vi "Get Name.vi"(8 "error in (no error)":errorcluster, 11 "Release in":refnum<class "Release.lvclass">) -> (0 "error out":errorcluster, 2 "Command Name":string, 3 "Release out":refnum<class "Release.lvclass">)   [LabVIEW 2014, in "Grabber.lvlib" / "Release.lvlib" / "Release.lvclass"]
uses:
  Release.lvclass
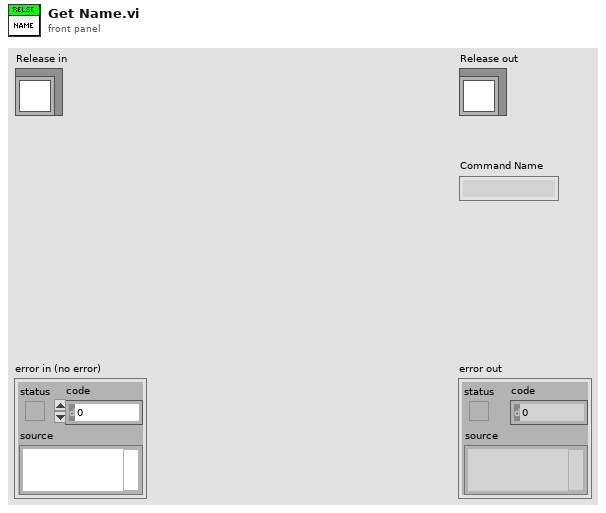
[diagram p1: front panel]
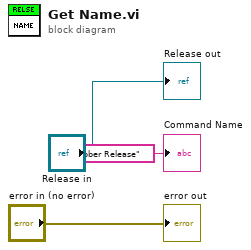
[diagram p0: block diagram]
diagram:
  "error out" <- "error in (no error)"
  "Release out" <- "Release in"
  "Command Name" <- "Grabber Release" ("Command Name")
